vi "RichToFlatnixnet_grpc_LinCommResponse.vi"(5 "OutputClusterType":T1, 11 "InputCluster":T3) -> (3 "OutputCluster":T1)   [LabVIEW 2025, in "grpc-xnet_client.lvlib"]
uses:
  nixnet_grpc_LinCommResponse.ctl
  nixnet_grpc_LinCommState.ctl
  nixnet_grpc_LinCommResponse_Flat.ctl
  grpc-xnet_client.lvlib
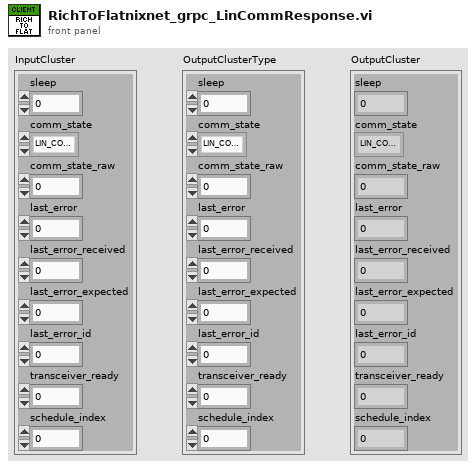
[diagram p1: front panel]
types:
  T1 = typedef "grpc-xnet_client.lvlib/nixnet_grpc_LinCommResponse_Flat.ctl" = cluster{"sleep":u32, "comm_state":T2, "comm_state_raw":u32, "last_error":u32, "last_error_received":u32, "last_error_expected":u32, "last_error_id":u32, "transceiver_ready":u32, "schedule_index":u32}
  T2 = typedef "grpc-xnet_client.lvlib/nixnet_grpc_LinCommState.ctl" = enum32{"LIN_COMM_STATE_IDLE", "LIN_COMM_STATE_ACTIVE", "LIN_COMM_STATE_INACTIVE"}
  T3 = typedef "grpc-xnet_client.lvlib/nixnet_grpc_LinCommResponse.ctl" = cluster{"sleep":u32, "comm_state":T2, "comm_state_raw":u32, "last_error":u32, "last_error_received":u32, "last_error_expected":u32, "last_error_id":u32, "transceiver_ready":u32, "schedule_index":u32}
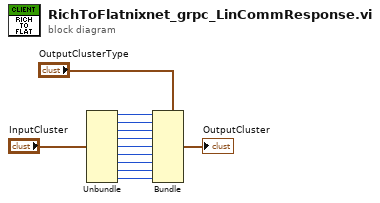
[diagram p0: block diagram]
diagram:
  n1 = Unbundle "Unbundle"("InputCluster") -> ("sleep"=w9:u32, "comm_state"=w8:T2, "comm_state_raw"=w7:u32, "last_error"=w6:u32, "last_error_received"=w5:u32, "last_error_expected"=w4:u32, "last_error_id"=w3:u32, "transceiver_ready"=w2:u32, "schedule_index"=w1:u32)
  n2 = Bundle "Bundle"(cluster="OutputClusterType", "sleep"=w9, "comm_state"=w8, "comm_state_raw"=w7, "last_error"=w6, "last_error_received"=w5, "last_error_expected"=w4, "last_error_id"=w3, "transceiver_ready"=w2, "schedule_index"=w1) -> (→"OutputCluster":T1)
